vi "abas.vi"() -> ()   [LabVIEW 2018]
panel:
  in  "Tab Control":T1(tab)
  in  "Iniciar teste":bool
  in  "Próximo passo - Pressão":bool
  out "Temperatura":dbl
  out "Thermometer":dbl(slide) scale=0.0..100.0
  in  "Próximo passo - Resultados":bool
  out "Reprovado":bool
  out "Aprovado":bool
  out "Gauge":dbl(knob) scale=0.0..100.0
  out "Pressão":dbl
  in  "Reiniciar":bool
  out "Boolean 5":bool
  out "Boolean 6":bool
  out "Pressão":dbl
  out "Temperatura":dbl
  out "Boolean 4":bool
  out "Boolean 3":bool
  out "Boolean 2":bool
  out "Boolean":bool
  # "Novo teste ->"
  # "Teste de temperatura e pressão."
  # "Coloque a amostra no dispositivo de teste.\n\n\nQuando o resultado aparecer, pressione no botão \"PRÓXIMO PASSO\"."
  # "Teste de temperatura"
  # "Teste de pressão"
  # "Aprovado"
  # "Reprovado"
  # "Temperatura"
  # "Pressão"
  # "Final"
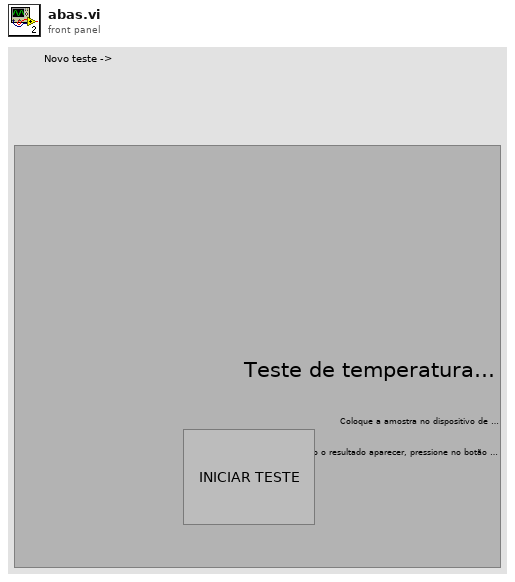
[diagram p1: front panel]
types:
  T1 = enum32{"Início", "Temperatura", "Pressão", "Resultados"}
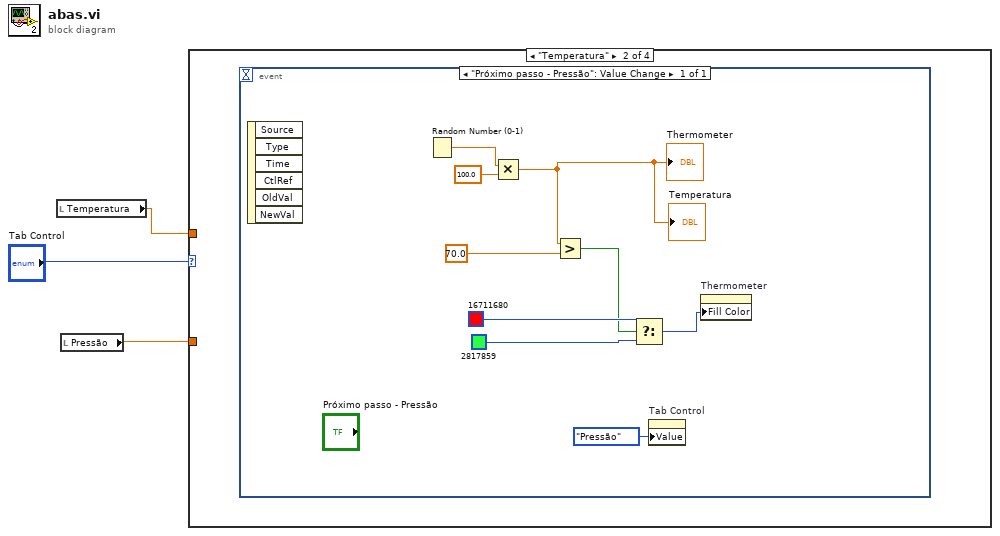
[diagram p0: block diagram]
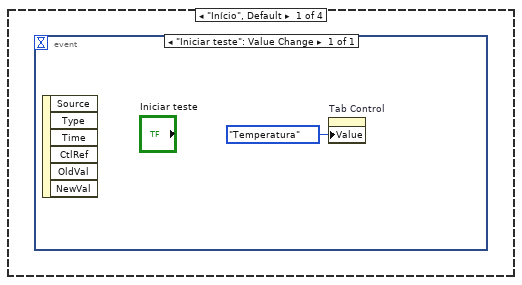
[diagram p2: hidden frame]
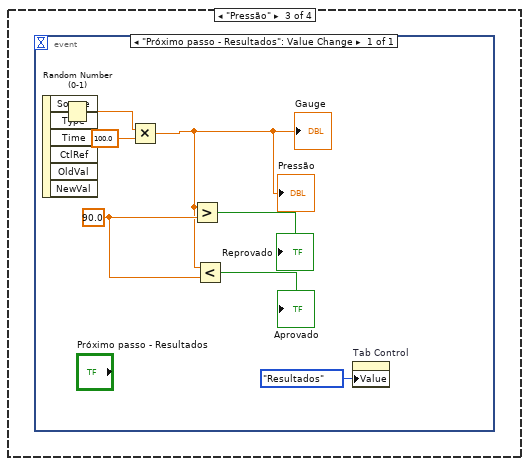
[diagram p3: hidden frame]
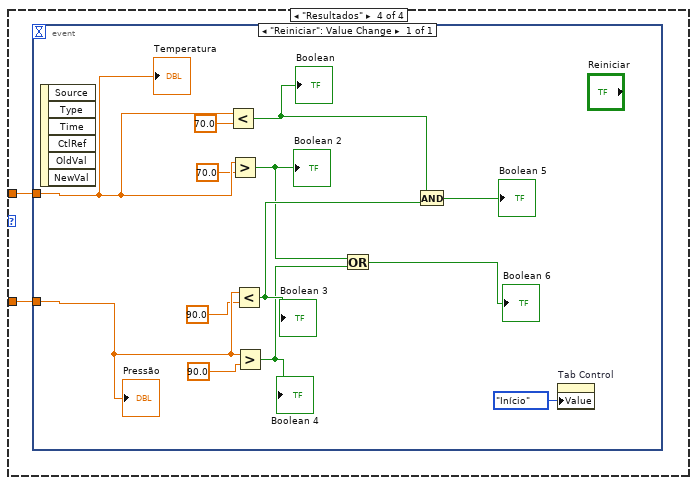
[diagram p4: hidden frame]
diagram:
  n1 = local read "Temperatura"() -> (w2:dbl)
  n2 = local read "Pressão"() -> (w1:dbl)
  n3 = case shown="\"Temperatura\"" "Tab Control" {
    tunnel: w2 -> [_ _ _ w21]
    tunnel: w1 -> [_ _ _ w22]
    frame "Início", Default {
      n4 = event shown="[0] \"Iniciar teste\": Value Change" {
        selector: _ -> [_]
        dyn-events: _ -> [_]
        timeout: _ -> [_]
        event "Iniciar teste": Value Change {
          n5 = event-data() -> ()  [unwired: 1 in, 6 out]
          n6 = property on="Tab Control" class="TabCtl (strict)"("Value"=T1."Temperatura" ("Tab Control")) -> ()  [unwired: 2 in, 2 out]
        }
      }
    }
    frame "Temperatura" {
      n7 = event shown="[0] \"Próximo passo - Pressão\": Value Change" {
        selector: _ -> [_]
        dyn-events: _ -> [_]
        timeout: _ -> [_]
        event "Próximo passo - Pressão": Value Change {
          n8 = event-data() -> ()  [unwired: 1 in, 6 out]
          n9 = Random Number (0-1)() -> (number: 0 to 1=w11:dbl)
          n10 = Multiply(x=w11, y=100.0) -> (x*y=w5:dbl)
          "Thermometer" <- w5
          "Temperatura" <- w5
          n11 = Greater?(x=w5, y=70.0) -> (0:w6:bool)
          n12 = Select(t=u32 16711680, s=w6, f=u32 2817859) -> (s? t:f=w7:u32)
          n13 = property on="Tab Control" class="TabCtl (strict)"("Value"=T1."Pressão" ("Tab Control")) -> ()  [unwired: 2 in, 2 out]
          n14 = property on="Thermometer" class="Slide (strict)"("Fill Color"=w7) -> ()  [unwired: 2 in, 2 out]
        }
      }
    }
    frame "Pressão" {
      n15 = event shown="[0] \"Próximo passo - Resultados\": Value Change" {
        selector: _ -> [_]
        dyn-events: _ -> [_]
        timeout: _ -> [_]
        event "Próximo passo - Resultados": Value Change {
          w17 = 90.0 ("y")
          n16 = event-data() -> ()  [unwired: 1 in, 6 out]
          n17 = Random Number (0-1)() -> (number: 0 to 1=w19:dbl)
          n18 = Multiply(x=w19, y=100.0) -> (x*y=w16:dbl)
          "Pressão" <- w16
          "Gauge" <- w16
          n19 = Greater?(x=w16, y=w17) -> (0:→"Reprovado":bool)
          n20 = Less?(x=w16, y=w17) -> (x < y?=→"Aprovado":bool)
          n21 = property on="Tab Control" class="TabCtl (strict)"("Value"=T1."Resultados" ("Tab Control")) -> ()  [unwired: 2 in, 2 out]
        }
      }
    }
    frame "Resultados" {
      n22 = event shown="[0] \"Reiniciar\": Value Change" {
        selector: _ -> [_]
        dyn-events: _ -> [_]
        timeout: _ -> [_]
        tunnel: w22 -> [w35]
        tunnel: w21 -> [w34]
        event "Reiniciar": Value Change {
          n23 = event-data() -> ()  [unwired: 1 in, 6 out]
          n24 = Less?(x=w34, y=70.0) -> (x < y?=w29:bool)
          "Boolean" <- w29
          n25 = Greater?(x=w34, y=70.0) -> (0:w25:bool)
          "Boolean 2" <- w25
          n26 = Less?(x=w35, y=90.0) -> (x < y?=w28:bool)
          "Boolean 3" <- w28
          n27 = Greater?(x=w35, y=90.0) -> (0:w26:bool)
          "Boolean 4" <- w26
          n28 = Or(x=w25, y=w26) -> (x .or. y?=→"Boolean 6":bool)
          n29 = And(x=w29, y=w28) -> (x .and. y?=→"Boolean 5":bool)
          n30 = property on="Tab Control" class="TabCtl (strict)"("Value"=T1."Início" ("Tab Control")) -> ()  [unwired: 2 in, 2 out]
          "Temperatura" <- w34
          "Pressão" <- w35
        }
      }
    }
  }
